vi "Get BLISS_Rand Between (I32 Inclusive).vi"(10 "lo limit (I32 inclusive)":i32, 11 "hi limit (I32 inclusive)":i32) -> (3 "Result":i32)   [LabVIEW 2020]
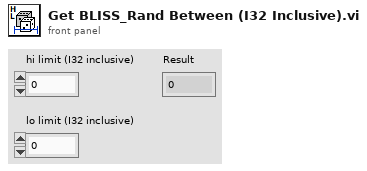
[diagram p1: front panel]
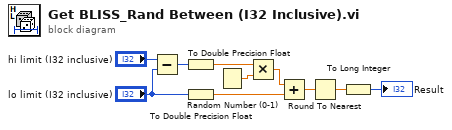
[diagram p0: block diagram]
diagram:
  n1 = Subtract(x="hi limit (I32 inclusive)", y="lo limit (I32 inclusive)") -> (x-y=w3:i32)
  n2 = To Double Precision Float(number=w3) -> (double precision float=w4:dbl)
  n3 = To Double Precision Float(number="lo limit (I32 inclusive)") -> (double precision float=w7:dbl)
  n4 = Random Number (0-1)() -> (number: 0 to 1=w5:dbl)
  n5 = Multiply(x=w4, y=w5) -> (x*y=w6:dbl)
  n6 = Add(x=w6, y=w7) -> (x+y=w2:dbl)
  n7 = Round To Nearest(number=w2) -> (nearest integer value=w8:dbl)
  n8 = To Long Integer(number=w8) -> (32bit integer=→"Result":i32)
